vi "HIL_Query.vi"(0 "System no.":i32=1 min=1 max=4 step=1, 2 "DeviceID to query":i32[](array[numeric]), 3 "DeviceLED":i32[](array[numeric]), 4 "All DeviceIDs?":bool, 5 "error in":errorcluster) -> (14 "State":i32[](array[numeric]), 16 "Queried DeviceIDs out":i32[](array[numeric]), 17 "DeviceLED out":i32[](array[numeric]), 19 "error out":errorcluster)   [LabVIEW 2020]
doc: "Returns the state of the LEDs of a Human Interface Device (HID). \"LED\" stands for hardware-dependent output, which can be an LED or a force-feedback actuator. See controller user manual for details."
uses:
  Global1.vi
panel:
  # "Returns the state of the LEDs of a Human Interface Device (HID). \"LED\" stands for \nhardware-dependent output, which can be an LED or a force-feedback actuator. See \ncontroller User Manual for details."
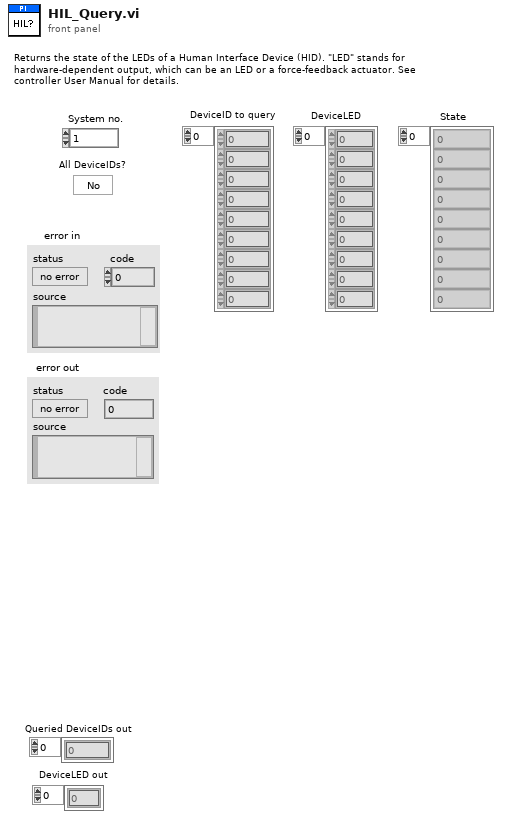
[diagram p1: front panel]
types:
  T1 = typedef "Syntax.ctl" = enum16{"GCS 1.0", "GCS 2.0", "GCS 3.0"}
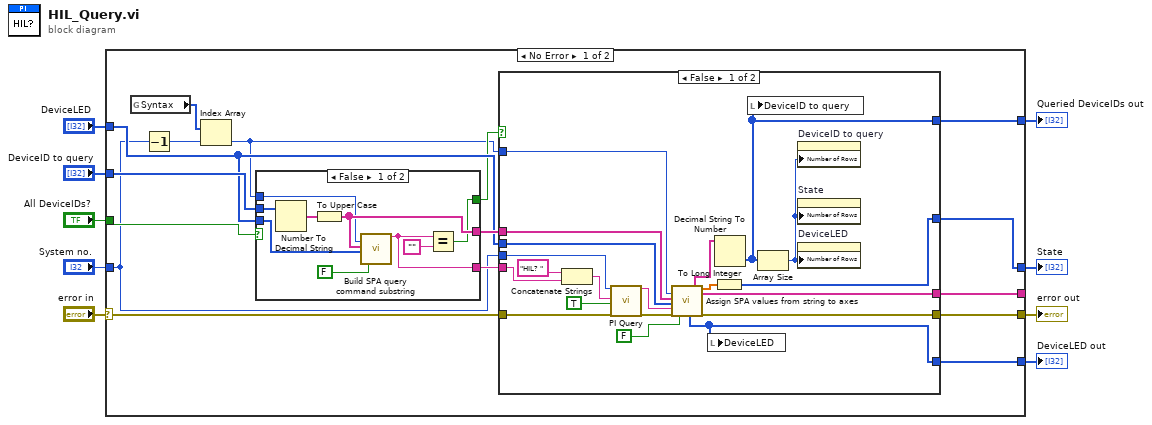
[diagram p0: block diagram]
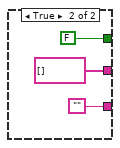
[diagram p2: hidden frame]
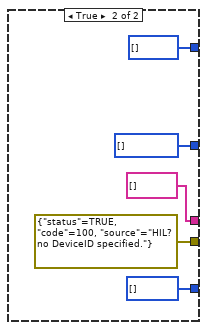
[diagram p3: hidden frame]
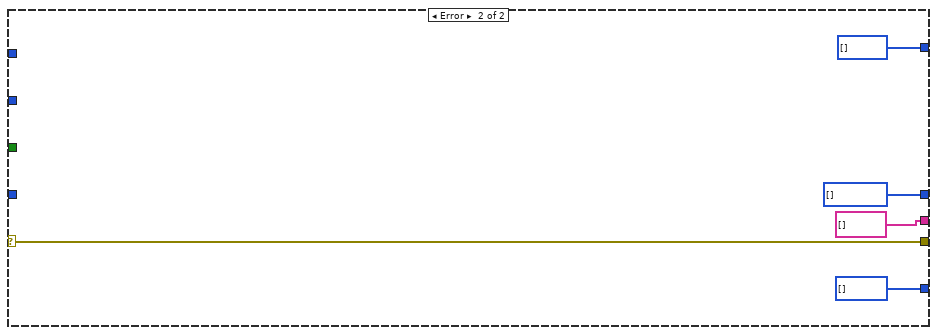
[diagram p4: hidden frame]
diagram:
  n1 = case shown="No Error" "error in" {
    selector: "error in" -> [w10 w63]
    tunnel: "DeviceID to query" -> [w25 _]
    tunnel: "System no." -> [w14 _]
    tunnel: "DeviceLED" -> [w22 _]
    tunnel: [w21 w63] -> w6
    tunnel: [w19 i32[] [] ("Parameter values")] -> w5
    tunnel: "All DeviceIDs?" -> [w18 _]
    tunnel: [w17 string[] [] ("Parameter strings")] -> _
    tunnel: [w12 i32[] [] ("Queried axes out")] -> w3
    tunnel: [w11 i32[] [] ("Parameter no. out")] -> w2
    frame No Error {
      n2 = global read "Global1.vi" "Syntax"() -> (w15:T1[])
      n3 = Decrement(x=w14) -> (x-1=w16:i32)
      n4 = Index Array(array=w15, index=w16) -> (element=w13:T1)
      n5 = case shown="False" w18 {
        tunnel: w25 -> [w27 _]
        tunnel: [w34 "" ("Command substring")] -> w24
        tunnel: [w33 string[] [] ("Designator to query")] -> w23
        tunnel: w22 -> [w32 _]
        tunnel: [w31 FALSE] -> w20
        tunnel: w13 -> [w30 _]
        frame False {
          n6 = Number To Decimal String(number=w27) -> (decimal integer string=w26:string[])  [unwired: 1 out]
          n7 = To Upper Case(1:w26) -> (0:w33:string[])
          n8 = call "Build SPA query command substring.vi"("Syntax"=w30, "Axes to query"=w33, "Parameter number"=w32, "Parameter no. format \n(Decimal: FALSE)"=FALSE ("Parameter no. format \n(Decimal: FALSE)")) -> ("Command substring"=w34:string)  [unwired: 3 in, 12 out]
          n9 = Equal?(x=w34, y="" ("x")) -> (x = y?=w31:bool)
        }
        frame True {
        }
      }
      n10 = case shown="False" w20 {
        tunnel: w10 -> [w49 _]
        tunnel: w24 -> [w54 _]
        tunnel: w23 -> [w53 _]
        tunnel: w14 -> [w42 _]
        tunnel: w22 -> [w52 _]
        tunnel: [w38 errorcluster {"status"=TRUE, "code"=100, "source"="HIL? no DeviceID specified."} ("error out")] -> w21
        tunnel: [w41 i32[] [] ("Parameter values")] -> w19
        tunnel: [w50 string[] [] ("Parameter strings")] -> w17
        tunnel: w13 -> [w48 _]
        tunnel: [w44 i32[] [] ("Queried axes out")] -> w12
        tunnel: [w47 i32[] [] ("Parameter no. out")] -> w11
        frame False {
          n11 = Concatenate Strings("HIL? ", w54) -> (w55:string)
          n12 = call "PI Query.vi"("System no."=w42, "String to send"=w55, "Attach termination char.?"=TRUE ("Attach Linefeed?"), "error in"=w49) -> ("String read"=w39:string, "error out"=w40:errorcluster)  [unwired: 3 in, 11 out]
          n13 = call "Assign SPA values from string to axes.vi"("Syntax"=w48, "Queried axes"=w53, "Parameter no."=w52, "Input string"=w39, "error in"=w40, "Parameter no. format \n(Decimal: FALSE)"=FALSE ("Parameter no. format \n(Decimal: FALSE)")) -> ("Parameter no. out"=w47:i32[], "Queried axes out"=w45:string[], "Parameter values"=w51:dbl[], "Parameter strings"=w50:string[], "error out"=w38:errorcluster)  [unwired: 2 in, 7 out]
          n14 = local write "DeviceLED"(w47) -> ()
          n15 = To Long Integer(number=w51) -> (32bit integer=w41:i32[])
          n16 = Decimal String To Number(string=w45) -> (number=w44:i32[])  [unwired: 3 out]
          n17 = local write "DeviceID to query"(w44) -> ()
          n18 = Array Size(array=w44) -> (size(s)=w46:i32)
          n19 = property on="DeviceID to query" class="Arr (strict)"("Number of Rows"=w46) -> ()  [unwired: 2 in, 2 out]
          n20 = property on="State" class="Arr (strict)"("Number of Rows"=w46) -> ()  [unwired: 2 in, 2 out]
          n21 = property on="DeviceLED" class="Arr (strict)"("Number of Rows"=w46) -> ()  [unwired: 2 in, 2 out]
        }
        frame True {
        }
      }
    }
    frame Error {
    }
  }
  "error out" <- w6
  "State" <- w5
  "Queried DeviceIDs out" <- w3
  "DeviceLED out" <- w2
